vi "NEVSTOP-Programming-Palette-API.vi"   [LabVIEW 2017]
doc: "Aggregates the utility VIs used by the palette's own tooling, coordinating the application, file and front-panel helpers behind one diagram."
uses:
  3ba386b1-cb53-471e-a5a6-b63e9b742c3e.vi
  48ac784f-7277-43a7-9ce3-f6934932dccd.vi
  b4569d0b-a93e-4555-bf83-1b6fe347ea94.vi
  Configuration/ClusterCfgTable/ClusterCfgTable.lvlib
  d6c0909c-03a2-4aab-83df-012d95666977.vi
  745de1ed-1428-40df-89db-6cab81be991d.vi
  Configuration/ClusterCfgTable/_instance/_Replace Configuration Table By ID(Element).vi
  Configuration/Ini/ini_configuration.lvlib
  d1296e84-d1f0-49ac-bf24-d8d54a753f09.vi
  700570c2-d53b-4e56-866b-3bd389334478.vi
  a3570983-0c30-47b3-97b5-a3aa9e015edb.vi
  Synchronization/SyncStart/SyncStart.lvlib
  b01996f5-150f-489d-8173-70cda26021f9.vi
  e677bb68-a6b2-4e6c-8da2-4dd6df72fdad.vi
  String/_Support/DataType Cacher(Data).vi
  7718a973-84a2-4da4-9bf8-1d93d3cab6de.vi
  222cb87d-9eb1-48af-8acb-874464f7f130.vi
  43686ab0-ed57-4da5-a21a-759ef75a850b.vi
  Signal/_Instance/_Number Count Down(Element).vi
  945e71ae-735a-4d0d-bbb4-134247c600ba.vi
  d4d2297e-5f1e-45f2-ae9a-f9a58a24edbc.vi
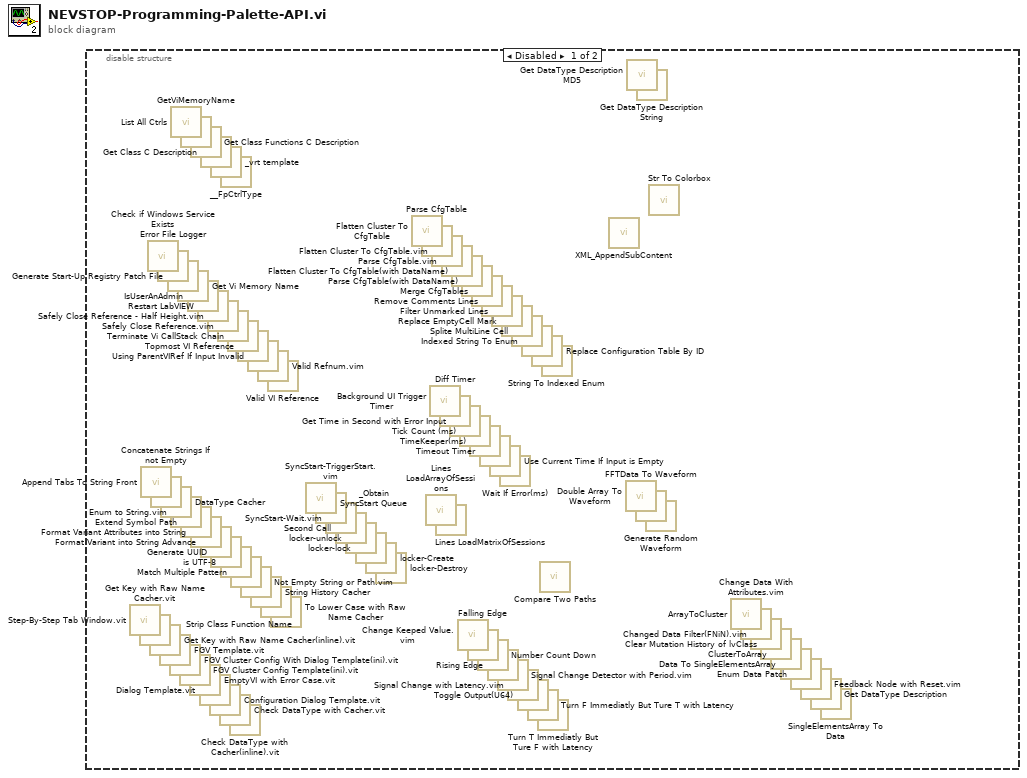
[diagram p0: block diagram]
diagram:
  n1 = disable-structure shown="Disabled" {
    frame Disabled {
      n2 = call "Step-By-Step Tab Window.vit"() -> ()  [unwired: 10 in, 2 out]
      n3 = call "Get Key with Raw Name Cacher.vit"() -> ()  [unwired: 9 in, 3 out]
      n4 = call "Append Tabs To String Front.vi"() -> ()  [unwired: 5 in, 1 out]
      n5 = call "Check if Windows Service Exists.vi"() -> ()  [unwired: 8 in, 4 out]
      n6 = call "Get Key with Raw Name Cacher(inline).vit"() -> ()  [unwired: 9 in, 3 out]
      n7 = call "Concatenate Strings If not Empty.vi"() -> ()  [unwired: 5 in, 1 out]
      n8 = call "Error File Logger.vi"() -> ()  [unwired: 14 in, 2 out]
      n9 = call "FGV Template.vit"() -> ()  [unwired: 10 in, 2 out]
      n10 = call-poly "DataType Cacher.vi"() -> ()  [unwired: 7 in, 5 out]
      n11 = call "Generate Start-Up Registry Patch File.vi"() -> ()  [unwired: 11 in, 1 out]
      n12 = call "FGV Cluster Config With Dialog Template(ini).vit"() -> ()  [unwired: 8 in, 4 out]
      n13 = call "List All Ctrls.vi"() -> ()  [unwired: 8 in, 4 out]
      n14 = call "Enum to String.vim"() -> ()  [unwired: 1 in, 1 out]
      n15 = call "Get Vi Memory Name.vi"() -> ()  [unwired: 9 in, 3 out]
      n16 = call "FGV Cluster Config Template(ini).vit"() -> ()  [unwired: 9 in, 3 out]
      n17 = call "GetViMemoryName.vi"() -> ()  [unwired: 9 in, 3 out]
      n18 = call "Extend Symbol Path.vi"() -> ()  [unwired: 3 in, 1 out]
      n19 = call "IsUserAnAdmin.vi"() -> ()  [unwired: 10 in, 2 out]
      n20 = call "EmptyVI with Error Case.vit"() -> ()  [unwired: 11 in, 1 out]
      n21 = call "Get Class Functions C Description.vi"() -> ()  [unwired: 10 in, 2 out]
      n22 = call "Format Variant Attributes into String.vi"() -> ()  [unwired: 10 in, 2 out]
      n23 = call "Restart LabVIEW.vi"() -> ()  [unwired: 1 in]
      n24 = call "Dialog Template.vit"() -> ()  [unwired: 11 in, 1 out]
      n25 = call "Get Class C Description.vi"() -> ()  [unwired: 10 in, 2 out]
      n26 = call "Format Variant into String Advance.vi"() -> ()  [unwired: 9 in, 3 out]
      n27 = call "Safely Close Reference - Half Height.vim"() -> ()  [unwired: 11 in, 1 out]
      n28 = call "Configuration Dialog Template.vit"() -> ()  [unwired: 11 in, 1 out]
      n29 = call "_vrt template.vi"() -> ()  [unwired: 11 in, 1 out]
      n30 = call "Generate UUID.vi"() -> ()  [unwired: 11 in, 1 out]
      n31 = call "Safely Close Reference.vim"() -> ()  [unwired: 11 in, 1 out]
      n32 = call "Check DataType with Cacher.vit"() -> ()  [unwired: 8 in, 4 out]
      n33 = call "__FpCtrlType.vi"() -> ()  [unwired: 8 in, 4 out]
      n34 = call "is UTF-8.vi"() -> ()  [unwired: 11 in, 1 out]
      n35 = call "Terminate Vi CallStack Chain.vi"() -> ()  [unwired: 12 in]
      n36 = call "Check DataType with Cacher(inline).vit"() -> ()  [unwired: 8 in, 4 out]
      n37 = call "Match Multiple Pattern.vi"() -> ()  [unwired: 7 in, 5 out]
      n38 = call "Topmost VI Reference.vi"() -> ()  [unwired: 5 in, 1 out]
      n39 = call "Not Empty String or Path.vim"() -> ()  [unwired: 1 in, 1 out]
      n40 = call "Using ParentVIRef If Input Invalid.vi"() -> ()  [unwired: 6 in, 2 out]
      n41 = call "String History Cacher.vi"() -> ()  [unwired: 11 in, 1 out]
      n42 = call "Valid Refnum.vim"() -> ()  [unwired: 3 in, 1 out]
      n43 = call "Strip Class Function Name.vi"() -> ()  [unwired: 3 in, 3 out]
      n44 = call "Valid VI Reference.vi"() -> ()  [unwired: 10 in, 1 out]
      n45 = call "To Lower Case with Raw Name Cacher.vi"() -> ()  [unwired: 9 in, 3 out]
      n46 = call "_Obtain SyncStart Queue.vi"() -> ()  [unwired: 10 in, 2 out]
      n47 = call "SyncStart-TriggerStart.vim"() -> ()  [unwired: 11 in, 1 out]
      n48 = call "SyncStart-Wait.vim"() -> ()  [unwired: 11 in, 1 out]
      n49 = call "Second Call.vi"() -> ()  [unwired: 1 out]
      n50 = call "locker-unlock.vi"() -> ()  [unwired: 10 in, 2 out]
      n51 = call "locker-lock.vi"() -> ()  [unwired: 10 in, 2 out]
      n52 = call "locker-Create.vi"() -> ()  [unwired: 10 in, 2 out]
      n53 = call "locker-Destroy.vi"() -> ()  [unwired: 11 in, 1 out]
      n54 = call "Flatten Cluster To CfgTable.vi"() -> ()  [unwired: 10 in, 2 out]
      n55 = call "Parse CfgTable.vi"() -> ()  [unwired: 9 in, 3 out]
      n56 = call "Lines LoadArrayOfSessions.vi"() -> ()  [unwired: 8 in, 4 out]
      n57 = call "Background UI Trigger Timer.vi"() -> ()  [unwired: 9 in, 3 out]
      n58 = call "Flatten Cluster To CfgTable.vim"() -> ()  [unwired: 9 in, 3 out]
      n59 = call "Lines LoadMatrixOfSessions.vi"() -> ()  [unwired: 9 in, 3 out]
      n60 = call "Diff Timer.vi"() -> ()  [unwired: 10 in, 2 out]
      n61 = call "Parse CfgTable.vim"() -> ()  [unwired: 10 in, 2 out]
      n62 = call "Get Time in Second with Error Input.vi"() -> ()  [unwired: 4 in, 2 out]
      n63 = call "Flatten Cluster To CfgTable(with DataName).vi"() -> ()  [unwired: 9 in, 3 out]
      n64 = call "Change Keeped Value.vim"() -> ()  [unwired: 11 in, 1 out]
      n65 = call "Tick Count (ms).vi"() -> ()  [unwired: 10 in, 2 out]
      n66 = call "Parse CfgTable(with DataName).vi"() -> ()  [unwired: 9 in, 3 out]
      n67 = call "Falling Edge.vi"() -> ()  [unwired: 11 in, 1 out]
      n68 = call "TimeKeeper(ms).vi"() -> ()  [unwired: 9 in, 3 out]
      n69 = call "Merge CfgTables.vi"() -> ()  [unwired: 10 in, 2 out]
      n70 = call-poly "Number Count Down.vi"() -> ()  [unwired: 8 in, 2 out]
      n71 = call "Timeout Timer.vi"() -> ()  [unwired: 8 in, 2 out]
      n72 = call "Remove Comments Lines.vi"() -> ()  [unwired: 10 in, 2 out]
      n73 = call "Rising Edge.vi"() -> ()  [unwired: 11 in, 1 out]
      n74 = call "Use Current Time If Input is Empty.vi"() -> ()  [unwired: 1 in, 1 out]
      n75 = call "Filter Unmarked Lines.vi"() -> ()  [unwired: 10 in, 2 out]
      n76 = call "Signal Change Detector with Period.vim"() -> ()  [unwired: 10 in, 2 out]
      n77 = call "Wait If Error(ms).vi"() -> ()  [unwired: 14 in, 2 out]
      n78 = call "Replace EmptyCell Mark.vi"() -> ()  [unwired: 10 in, 2 out]
      n79 = call "Signal Change with Latency.vim"() -> ()  [unwired: 10 in, 2 out]
      n80 = call "Splite MultiLine Cell.vi"() -> ()  [unwired: 10 in, 2 out]
      n81 = call "Toggle Output(U64).vi"() -> ()  [unwired: 11 in, 1 out]
      n82 = call "Indexed String To Enum.vi"() -> ()  [unwired: 10 in, 2 out]
      n83 = call "Turn F Immediatly But Ture T with Latency.vi"() -> ()  [unwired: 10 in, 2 out]
      n84 = call-poly "Replace Configuration Table By ID.vi"() -> ()  [unwired: 10 in, 2 out]
      n85 = call "Turn T Immediatly But Ture F with Latency.vi"() -> ()  [unwired: 10 in, 2 out]
      n86 = call <vilib>:"Compare Two Paths.vi"() -> ()  [unwired: 8 in, 4 out]
      n87 = call "String To Indexed Enum.vi"() -> ()  [unwired: 10 in, 2 out]
      n88 = call "XML_AppendSubContent.vi"() -> ()  [unwired: 11 in, 1 out]
      n89 = call "Double Array To Waveform.vi"() -> ()  [unwired: 11 in, 1 out]
      n90 = call "Get DataType Description MD5.vi"() -> ()  [unwired: 10 in, 2 out]
      n91 = call "FFTData To Waveform.vi"() -> ()  [unwired: 11 in, 1 out]
      n92 = call "Get DataType Description String.vi"() -> ()  [unwired: 10 in, 2 out]
      n93 = call "Generate Random Waveform.vi"() -> ()  [unwired: 10 in, 2 out]
      n94 = call "Str To Colorbox.vi"() -> ()  [unwired: 1 in, 1 out]
      n95 = call "ArrayToCluster.vi"() -> ()  [unwired: 10 in, 2 out]
      n96 = call "Change Data With Attributes.vim"() -> ()  [unwired: 10 in, 2 out]
      n97 = call "Changed Data Filter(FNiN).vim"() -> ()  [unwired: 8 in, 4 out]
      n98 = call "Clear Mutation History of lvClass.vi"() -> ()  [unwired: 10 in, 2 out]
      n99 = call "ClusterToArray.vi"() -> ()  [unwired: 10 in, 2 out]
      n100 = call "Data To SingleElementsArray.vi"() -> ()  [unwired: 8 in, 4 out]
      n101 = call "Enum Data Patch.vi"() -> ()  [unwired: 10 in, 2 out]
      n102 = call "Feedback Node with Reset.vim"() -> ()  [unwired: 7 in, 1 out]
      n103 = call-poly "Get DataType Description.vi"() -> ()  [unwired: 10 in, 2 out]
      n104 = call "SingleElementsArray To Data.vi"() -> ()  [unwired: 10 in, 2 out]
    }
    frame Enabled {
    }
  }
